vi "Assignment2_3.vi"() -> ()   [LabVIEW 2025]
doc: "This VI calculates the time (sec) of LED in which it is turned ON, for various mechanical action of switch."
panel:
  out "Time (Sec) 6":i32
  out "Time (Sec) 5":i32
  out "Time (Sec) 4":i32
  out "Time (Sec) 3":i32
  out "Time (Sec) 2":i32
  out "Time (Sec)":i32
  out "LED 6":bool
  out "LED 5":bool
  out "LED 4":bool
  out "LED 3":bool
  out "LED 2":bool
  out "LED 1":bool
  in  "STOP":bool
  in  "RESET":bool
  in  "Latch Until Released":bool
  in  "Latch When Released":bool
  in  "Latch When Pressed":bool
  in  "Switch Until Released":bool
  in  "Switch When Released":bool
  in  "Switch When Pressed":bool
  # "INSTRUCTIONS:"
  # "1) Press \"RESET\" button to reset the values of all the timers to zero.\n2) Press \"STOP\" button to stop the program."
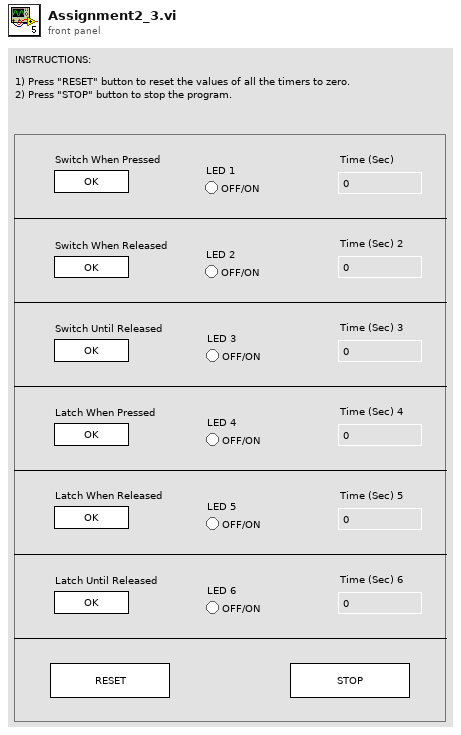
[diagram p1: front panel]
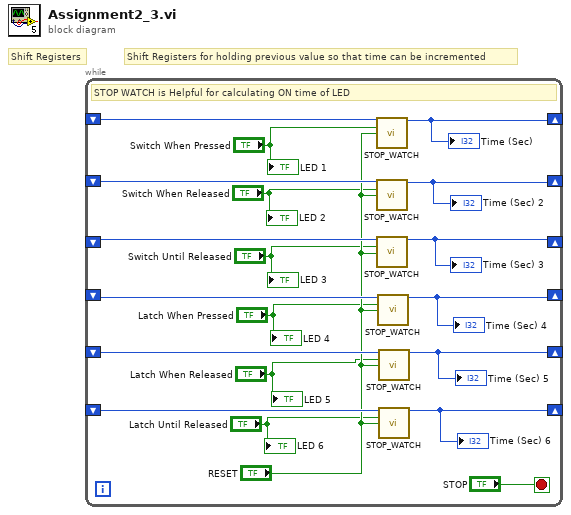
[diagram p0: block diagram]
diagram:
  # "Shift Registers"
  # "Shift Registers for holding previous value so that time can be incremented"
  n1 = while {
    shift-right: [w17] -> _
    shift-left: _ -> [w19]
    shift-right: [w11] -> _
    shift-left: _ -> [w16]
    shift-right: [w10] -> _
    shift-left: _ -> [w15]
    shift-right: [w9] -> _
    shift-left: _ -> [w14]
    shift-right: [w8] -> _
    shift-left: _ -> [w13]
    shift-right: [w7] -> _
    shift-left: _ -> [w12]
    stop <- "STOP" stop-if-true
    # "STOP WATCH is Helpful for calculating ON time of LED"
    n2 = call "STOP_WATCH.vi"("Variable"=w19, "Switch"="Switch When Pressed", "RESET"="RESET") -> ("Time (Sec)"=w17:i32)  [unwired: 12 in]
    "Time (Sec)" <- w17
    n3 = call "STOP_WATCH.vi"("Variable"=w16, "Switch"="Switch When Released", "RESET"="RESET") -> ("Time (Sec)"=w11:i32)  [unwired: 12 in]
    "Time (Sec) 2" <- w11
    n4 = call "STOP_WATCH.vi"("Variable"=w15, "Switch"="Switch Until Released", "RESET"="RESET") -> ("Time (Sec)"=w10:i32)  [unwired: 12 in]
    "Time (Sec) 3" <- w10
    n5 = call "STOP_WATCH.vi"("Variable"=w14, "Switch"="Latch When Pressed", "RESET"="RESET") -> ("Time (Sec)"=w9:i32)  [unwired: 12 in]
    "Time (Sec) 4" <- w9
    n6 = call "STOP_WATCH.vi"("Variable"=w13, "Switch"="Latch When Released", "RESET"="RESET") -> ("Time (Sec)"=w8:i32)  [unwired: 12 in]
    "Time (Sec) 5" <- w8
    n7 = call "STOP_WATCH.vi"("Variable"=w12, "Switch"="Latch Until Released", "RESET"="RESET") -> ("Time (Sec)"=w7:i32)  [unwired: 12 in]
    "Time (Sec) 6" <- w7
    "LED 1" <- "Switch When Pressed"
    "LED 2" <- "Switch When Released"
    "LED 3" <- "Switch Until Released"
    "LED 4" <- "Latch When Pressed"
    "LED 5" <- "Latch When Released"
    "LED 6" <- "Latch Until Released"
  }
